vi "Main.vi"() -> ()   [LabVIEW 2018] (continued)
            n624 = Index Array(array=w4544, index (row)=w4543, index (col)=w4543) -> (element=w4542:string)
            n625 = Equal?(x=w4542, y="T") -> (x = y?=w4540:bool)
            n626 = local read "ST102数据"() -> (w4537:string[])
            n627 = case shown="真" w4540 {
              tunnel: w4537 -> [w4577 w4583]
              tunnel: [w4573 w4580] -> w4552
              tunnel: w4536 -> [w4572 w4582]
              tunnel: w4545 -> [w4571 w4581]
              tunnel: w4539 -> [w4570 w4594]
              tunnel: w4538 -> [w4569 w4593]
              tunnel: [w4567 w4579] -> w4534
              frame False {
                n628 = call "SQL_Update.vi"("查询语句"=w4571, "表名"="Online", "error in (no error)"=w4569, "列名对应的值"=w4577, "列名"=string[] ["Last_Station", "Last_Result", "ST10_R_Date", "ST10_R_Time", "ST10_Result", "ST10_Pressure_Final", "ST10_Pressure_Upper", "ST10_Pressure_Lower", "ST10_Displacement_Final", "ST10_Displacement_Upper", "ST10_Displacement_Lower", "ST10_Inflextion_Point", "ST10_Inflextion_Point_Upper", "ST10_Inflextion_Point_Lower", "Grade", "ST10_Sleeve_5020001", "ST10_Flange_5025570"], "connection reference"=w4570) -> ("error out"=w4573:errorcluster)  [unwired: 4 in, 1 out]
                n629 = Unbundle By Name(w4573) -> ("status"=w4576:bool)
                n630 = Equal?(x=w4572, y="") -> (x = y?=w4574:bool)
                n631 = Or(x=w4576, y=w4574) -> (x .or. y?=w4567:bool)
              }
              frame True {
                w4589 = 0 ("索引 (行)")
                n632 = call "SQL_Select.vi"("要读取的列名"=string[] ["[102]"], "表名"="Rework_List", "error in (no error)"=w4593, "查询语句"=w4581, "查询条件"=TRUE, "connection reference"=w4594) -> ("error out"=w4584:errorcluster, "数据"=w4590:string[][], "connection reference out"=w4585:T5)  [unwired: 3 in]
                n633 = Index Array(array=w4590, index (row)=w4589, index (col)=w4589) -> (element=w4588:string)
                n634 = Equal?(x=w4588, y="T") -> (x = y?=w4586:bool)
                n635 = case shown="假" w4586 {
                  tunnel: w4585 -> [w4602 w4618]
                  tunnel: w4584 -> [w4603 w4617]
                  tunnel: w4583 -> [w4601 w4624]
                  tunnel: w4582 -> [w4598 w4619]
                  tunnel: w4581 -> [w4600 w4611]
                  tunnel: [w4599 w4610] -> w4580
                  tunnel: [w4596 w4608] -> w4579
                  frame False {
                    n636 = call "SQL_Update.vi"("查询语句"=w4600, "表名"="Online", "error in (no error)"=w4603, "列名对应的值"=w4601, "列名"=string[] ["Last_Station", "Last_Result", "ST10_R_Date", "ST10_R_Time", "ST10_Result", "ST10_Pressure_Final", "ST10_Pressure_Upper", "ST10_Pressure_Lower", "ST10_Displacement_Final", "ST10_Displacement_Upper", "ST10_Displacement_Lower", "ST10_Inflextion_Point", "ST10_Inflextion_Point_Upper", "ST10_Inflextion_Point_Lower", "Grade", "ST10_Sleeve_5020001", "ST10_Flange_5025570"], "connection reference"=w4602) -> ("error out"=w4599:errorcluster)  [unwired: 4 in, 1 out]
                    n637 = Unbundle By Name(w4599) -> ("status"=w4606:bool)
                    n638 = Equal?(x=w4598, y="") -> (x = y?=w4604:bool)
                    n639 = Or(x=w4606, y=w4604) -> (x .or. y?=w4596:bool)
                  }
                  frame True {
                    n640 = Delete From Array(array=w4624, length=2 ("长度"), index=0 ("索引")) -> (deleted portion=w4612:string[], array with subset deleted=w4621:string[])
                    n641 = call "SQL_Update.vi"("查询语句"=w4611, "表名"="Online", "error in (no error)"=w4617, "列名对应的值"=w4612, "列名"=string[] ["Last_Station", "Last_Result"], "connection reference"=w4618) -> ("error out"=w4616:errorcluster, "connection reference 2"=w4615:T5)  [unwired: 4 in]
                    n642 = call "SQL_Update.vi"("查询语句"=w4611, "表名"="Rework", "error in (no error)"=w4616, "列名对应的值"=w4621, "列名"=string[] ["ST10_R_Date", "ST10_R_Time", "ST10_Result", "ST10_Pressure_Final", "ST10_Pressure_Upper", "ST10_Pressure_Lower", "ST10_Displacement_Final", "ST10_Displacement_Upper", "ST10_Displacement_Lower", "ST10_Inflextion_Point", "ST10_Inflextion_Point_Upper", "ST10_Inflextion_Point_Lower", "Grade", "ST10_Sleeve_5020001", "ST10_Flange_5025570"], "connection reference"=w4615) -> ("error out"=w4610:errorcluster)  [unwired: 4 in, 1 out]
                    n643 = Unbundle By Name(w4610) -> ("status"=w4626:bool)
                    n644 = Equal?(x="", y=w4619) -> (x = y?=w4625:bool)
                    n645 = Or(x=w4626, y=w4625) -> (x .or. y?=w4608:bool)
                  }
                }
              }
            }
            n646 = case shown="假" w4534 {
              frame False {
                n647 = property on="ST10画曲线" class="Bool (严格)"("Val(Sgnl)"=TRUE ("值(信号)")) -> ()  [unwired: 2 in, 2 out]
              }
              frame True {
                n648 = local write "102数据回复写入"(TRUE ("102数据回复写入")) -> ()
                "数据保存请求回复102" <- "2" ("数据保存请求回复102")
              }
            }
            n649 = Delete From Array(array=w4537, length=2 ("长度"), index=0 ("索引")) -> (array with subset deleted=w4555:string[])  [unwired: 1 out]
            n650 = Insert Into Array(array=w4555, index=3 ("索引"), new element=w4536) -> (w4553:string[])
            n651 = Insert Into Array(array=string[][] [] ("数组"), index (row)=0 ("索引 (行)"), new element=w4553) -> (w4558:string[][])  [unwired: 1 in]
            n652 = Transpose 2D Array(2D array=w4558) -> (transposed array=w4535:string[][])
            n653 = property on="ST102_DATA" class="MCListbox (严格)"("ItemNames"=w4535) -> ()  [unwired: 2 in, 2 out]
            "ST102数据读取（事件）" <- FALSE ("ST10数据读取（事件）")
          }
          event "ST201扫码请求(事件)": Value Change {
            w4629 = path "D:/op201" ("路径")
            n654 = event-data() -> ()  [unwired: 1 in, 1 out]
            n655 = List Folder(path=w4629) -> (filenames=w4628:string[])  [unwired: 3 in, 3 out]
            n656 = for {
              tunnel: w4628 -> [w4660] mode=indexing
              tunnel: w4629 -> [w4661]
              n657 = Build Path(base path=w4661, name or relative path=w4660) -> (appended path=w4658:path)
              n658 = Delete(path (use dialog)=w4658, entire hierarchy (F)=TRUE ("整个层次结构(F)")) -> ()  [unwired: 3 in, 3 out]
            }
            n659 = local read "201二维码"() -> (w4634:string)
            n660 = Concatenate Strings("Where QRCode='" ("查询语句"), w4634, "'" ("字符串")) -> (w4651:string)
            n661 = call "SQL_Select.vi"("要读取的列名"=string[] ["Last_Station", "Last_Result"], "表名"="Online", "error in (no error)"=w4640, "查询语句"=w4651, "查询条件"=TRUE, "connection reference"=w4639) -> ("error out"=w4637:errorcluster, "数据"=w4650:string[][])  [unwired: 3 in, 1 out]
            n662 = case shown="无错误" w4637 {
              tunnel: w4650 -> [w4669 _]
              tunnel: ["1" ("右扫码请求回复") "2" ("右扫码请求回复")] -> w4630
              tunnel: [w4664 w4671] -> w4633
              tunnel: [w4663 w4671] -> w4632
              tunnel: [TRUE TRUE] -> w4631
              frame No Error {
                n663 = Index Array(array=w4669, index (row)=0 ("索引 (行)")) -> (element=w4666:string[])  [unwired: 1 in]
                n664 = Index Array(array=w4666, index #1=0 ("索引 (行)")) -> (element #1=w4663:string, element #2=w4664:string)  [unwired: 1 in]
              }
              frame Error {
                w4671 = ""
              }
            }
            "上一站号 (201)" <- w4632
            "上一站结果 (201)" <- w4633
            "扫码请求回复201" <- w4630
            n665 = local write "201扫码回复写入"(w4631) -> ()
            n666 = Get Date/Time String(want seconds? (F)=TRUE ("需要秒？(F)")) -> (time string=w4647:string)  [unwired: 2 in, 1 out]
            n667 = Format Date/Time String(time format string (%c)="%Y-%m-%d" ("时间格式字符串(%c)")) -> (date/time string=w4648:string)  [unwired: 2 in]
            n668 = Insert Into Array(array=string[] [] ("数组"), index=0 ("索引"), new element #1=w4648, new element #2=w4647, new element #3=w4634) -> (w4644:string[])
            n669 = Insert Into Array(array=string[][] [] ("数组"), index (row)=0 ("索引 (行)"), new element=w4644) -> (w4641:string[][])  [unwired: 1 in]
            n670 = Transpose 2D Array(2D array=w4641) -> (transposed array=w4638:string[][])
            n671 = property on="ST201_DATA" class="MCListbox (严格)"("ItemNames"=w4638) -> ()  [unwired: 2 in, 2 out]
            "ST201扫码请求(事件)" <- FALSE ("ST20扫码请求(事件)")
          }
          event "ST201数据读取(事件)": Value Change {
            n672 = event-data() -> ()  [unwired: 1 in, 1 out]
            n673 = flat-sequence {
              tunnel: w4677 -> [w4682]
              tunnel: w4678 -> [w4683]
              tunnel: [w4683] -> w4675
              tunnel: [w4682] -> w4674
              tunnel: w4675 -> [w4689]
              tunnel: w4674 -> [w4688]
              tunnel: [w4687] -> w4673
              tunnel: [w4783] -> w4676
              tunnel: w4673 -> [w4783]
              frame #0 {
                "ST201保存中" <- TRUE
              }
              frame #1 {
                w4695 = 0 ("索引 (行)")
                n674 = local read "201二维码"() -> (w4686:string)
                n675 = Concatenate Strings("Where QRCode='" ("查询语句"), w4686, "'" ("字符串")) -> (w4697:string)
                n676 = call "SQL_Select.vi"("要读取的列名"=string[] ["Rework_Status"], "表名"="Online", "error in (no error)"=w4688, "查询语句"=w4697, "查询条件"=TRUE, "connection reference"=w4689) -> ("error out"=w4690:errorcluster, "数据"=w4696:string[][], "connection reference out"=w4691:T5)  [unwired: 3 in]
                n677 = Index Array(array=w4696, index (row)=w4695, index (col)=w4695) -> (element=w4694:string)
                n678 = Equal?(x=w4694, y="T") -> (x = y?=w4692:bool)
                n679 = local read "201数据"() -> (w4685:string[])
                n680 = case shown="真" w4692 {
                  tunnel: w4685 -> [w4725 w4733]
                  tunnel: [w4721 w4730] -> w4687
                  tunnel: w4686 -> [w4720 w4732]
                  tunnel: w4697 -> [w4719 w4731]
                  tunnel: w4691 -> [w4718 w4744]
                  tunnel: w4690 -> [w4717 w4743]
                  tunnel: [w4715 w4729] -> w4684
                  frame False {
                    n681 = call "SQL_Update.vi"("查询语句"=w4719, "表名"="Online", "error in (no error)"=w4717, "列名对应的值"=w4725, "列名"=string[] ["Last_Station", "Last_Result", "ST201_Date", "ST201_Time", "ST201_Result", "ST201_Oil_Pressure_Final", "ST201_Oil_Pressure_Upper", "ST201_Oil_Pressure_Lower", "ST201_Oil_Displacement_Final", "ST201_Oil_Displacement_Upper", "ST201_Oil_Displacement_Lower", "ST201_Oil_Inflexion_Force_Final", "ST201_Oil_Inflexion_Force_Upper", "ST201_Oil_Inflexion_Force_Lower", "ST201_Bearing_Pressure_Final", "ST201_Bearing_Pressure_Upper", "ST201_Bearing_Pressure_Lower", "ST201_Bearing_Displacement_Final", "ST201_Bearing_Displacement_Upper", "ST201_Bearing_Displacement_Lower", "ST201_Bearing_Inflexion_Force_Final", "ST201_Bearing_Inflexion_Force_Upper", "ST201_Bearing_Inflexion_Force_Lower"], "connection reference"=w4718) -> ("error out"=w4721:errorcluster)  [unwired: 4 in, 1 out]
                    n682 = Unbundle By Name(w4721) -> ("status"=w4724:bool)
                    n683 = Equal?(x=w4720, y="") -> (x = y?=w4722:bool)
                    n684 = Or(x=w4724, y=w4722) -> (x .or. y?=w4715:bool)
                    n685 = case shown="假" w4715 {
                      tunnel: ["1" ("数据保存请求回复") "2" ("数据保存请求回复")] -> _
                      frame False {
                      }
                      frame True {
                      }
                    }
                  }
                  frame True {
                    w4739 = 0 ("索引 (行)")
                    n686 = call "SQL_Select.vi"("要读取的列名"=string[] ["[201]"], "表名"="Rework_List", "error in (no error)"=w4743, "查询语句"=w4731, "查询条件"=TRUE, "connection reference"=w4744) -> ("error out"=w4734:errorcluster, "数据"=w4740:string[][], "connection reference out"=w4735:T5)  [unwired: 3 in]
                    n687 = Index Array(array=w4740, index (row)=w4739, index (col)=w4739) -> (element=w4738:string)
                    n688 = Equal?(x=w4738, y="T") -> (x = y?=w4736:bool)
                    n689 = case shown="假" w4736 {
                      tunnel: w4735 -> [w4752 w4770]
                      tunnel: w4734 -> [w4753 w4769]
                      tunnel: w4733 -> [w4751 w4776]
                      tunnel: w4732 -> [w4748 w4771]
                      tunnel: w4731 -> [w4750 w4762]
                      tunnel: [w4749 w4763] -> w4730
                      tunnel: [w4746 w4760] -> w4729
                      frame False {
                        (unwired) TRUE
                        n690 = call "SQL_Update.vi"("查询语句"=w4750, "表名"="Online", "error in (no error)"=w4753, "列名对应的值"=w4751, "列名"=string[] ["Last_Station", "Last_Result", "ST201_Date", "ST201_Time", "ST201_Result", "ST201_Oil_Pressure_Final", "ST201_Oil_Pressure_Upper", "ST201_Oil_Pressure_Lower", "ST201_Oil_Displacement_Final", "ST201_Oil_Displacement_Upper", "ST201_Oil_Displacement_Lower", "ST201_Oil_Inflexion_Force_Final", "ST201_Oil_Inflexion_Force_Upper", "ST201_Oil_Inflexion_Force_Lower", "ST201_Bearing_Pressure_Final", "ST201_Bearing_Pressure_Upper", "ST201_Bearing_Pressure_Lower", "ST201_Bearing_Displacement_Final", "ST201_Bearing_Displacement_Upper", "ST201_Bearing_Displacement_Lower", "ST201_Bearing_Inflexion_Force_Final", "ST201_Bearing_Inflexion_Force_Upper", "ST201_Bearing_Inflexion_Force_Lower"], "connection reference"=w4752) -> ("error out"=w4749:errorcluster)  [unwired: 4 in, 1 out]
                        n691 = Unbundle By Name(w4749) -> ("status"=w4756:bool)
                        n692 = Equal?(x=w4748, y="") -> (x = y?=w4754:bool)
                        n693 = Or(x=w4756, y=w4754) -> (x .or. y?=w4746:bool)
                        n694 = case shown="假" w4746 {
                          tunnel: ["1" ("数据保存请求回复") "2" ("数据保存请求回复")] -> _
                          frame False {
                          }
                          frame True {
                          }
                        }
                      }
                      frame True {
                        n695 = Delete From Array(array=w4776, length=2 ("长度"), index=0 ("索引")) -> (deleted portion=w4764:string[], array with subset deleted=w4773:string[])
                        n696 = call "SQL_Update.vi"("查询语句"=w4762, "表名"="Online", "error in (no error)"=w4769, "列名对应的值"=w4764, "列名"=string[] ["Last_Station", "Last_Result"], "connection reference"=w4770) -> ("error out"=w4768:errorcluster, "connection reference 2"=w4767:T5)  [unwired: 4 in]
                        n697 = call "SQL_Update.vi"("查询语句"=w4762, "表名"="Rework", "error in (no error)"=w4768, "列名对应的值"=w4773, "列名"=string[] ["ST201_Date", "ST201_Time", "ST201_Result", "ST201_Oil_Pressure_Final", "ST201_Oil_Pressure_Upper", "ST201_Oil_Pressure_Lower", "ST201_Oil_Displacement_Final", "ST201_Oil_Displacement_Upper", "ST201_Oil_Displacement_Lower", "ST201_Oil_Inflexion_Force_Final", "ST201_Oil_Inflexion_Force_Upper", "ST201_Oil_Inflexion_Force_Lower", "ST201_Bearing_Pressure_Final", "ST201_Bearing_Pressure_Upper", "ST201_Bearing_Pressure_Lower", "ST201_Bearing_Displacement_Final", "ST201_Bearing_Displacement_Upper", "ST201_Bearing_Displacement_Lower", "ST201_Bearing_Inflexion_Force_Final", "ST201_Bearing_Inflexion_Force_Upper", "ST201_Bearing_Inflexion_Force_Lower"], "connection reference"=w4767) -> ("error out"=w4763:errorcluster)  [unwired: 4 in, 1 out]
                        n698 = Unbundle By Name(w4763) -> ("status"=w4778:bool)
                        n699 = Equal?(x="", y=w4771) -> (x = y?=w4777:bool)
                        n700 = Or(x=w4778, y=w4777) -> (x .or. y?=w4760:bool)
                        n701 = case shown="真" w4760 {
                          tunnel: ["1" ("数据保存请求回复") "2" ("数据保存请求回复")] -> _
                          frame False {
                          }
                          frame True {
                          }
                        }
                      }
                    }
                  }
                }
                n702 = case shown="真" w4684 {
                  frame False {
                    n703 = property on="ST201画曲线" class="Bool (严格)"("Val(Sgnl)"=TRUE ("值(信号)")) -> ()  [unwired: 2 in, 2 out]
                  }
                  frame True {
                    n704 = local write "201数据回复写入"(TRUE ("201数据回复写入")) -> ()
                    "数据保存请求回复201" <- "2" ("数据保存请求回复201")
                  }
                }
                n705 = Delete From Array(array=w4685, length=2 ("长度"), index=0 ("索引")) -> (array with subset deleted=w4706:string[])  [unwired: 1 out]
                n706 = Insert Into Array(array=w4706, index=2 ("索引"), new element=w4686) -> (w4704:string[])
                n707 = Insert Into Array(array=string[][] [] ("数组"), index (row)=0 ("索引 (行)"), new element=w4704) -> (w4709:string[][])  [unwired: 1 in]
                n708 = Transpose 2D Array(2D array=w4709) -> (transposed array=w4703:string[][])
                n709 = property on="ST201_DATA" class="MCListbox (严格)"("ItemNames"=w4703) -> ()  [unwired: 2 in, 2 out]
              }
              frame #2 {
                n710 = local write "ST201保存中"(FALSE) -> ()
              }
            }
            "ST201数据读取(事件)" <- FALSE ("ST20数据读取(事件)")
          }
          event "ST202扫码请求(事件)": Value Change {
            w4786 = "——" ("字符串")
            w4793 = path "D:/op202" ("路径")
            n711 = event-data() -> ()  [unwired: 1 in, 2 out]
            n712 = local read "202二维码"() -> (w4790:string)
            n713 = List Folder(path=w4793) -> (filenames=w4792:string[])  [unwired: 3 in, 3 out]
            n714 = for {
              tunnel: w4792 -> [w4812] mode=indexing
              tunnel: w4793 -> [w4813]
              n715 = Build Path(base path=w4813, name or relative path=w4812) -> (appended path=w4810:path)
              n716 = Delete(path (use dialog)=w4810, entire hierarchy (F)=TRUE ("整个层次结构(F)")) -> ()  [unwired: 3 in, 3 out]
            }
            n717 = Concatenate Strings("Where QRCode='" ("查询语句"), w4790, "'" ("字符串")) -> (w4806:string)
            n718 = call "SQL_Select.vi"("要读取的列名"=string[] ["Last_Station", "Last_Result"], "表名"="Online", "error in (no error)"=w4797, "查询语句"=w4806, "查询条件"=TRUE, "connection reference"=w4798) -> ("error out"=w4804:errorcluster, "数据"=w4805:string[][])  [unwired: 3 in, 1 out]
            n719 = case shown="无错误" w4804 {
              tunnel: w4805 -> [w4821 _]
              tunnel: ["1" ("右扫码请求回复") "2" ("右扫码请求回复")] -> w4787
              tunnel: [w4816 w4823] -> w4788
              tunnel: [w4815 w4823] -> w4789
              tunnel: [TRUE TRUE] -> w4796
              frame No Error {
                n720 = Index Array(array=w4821, index (row)=0 ("索引 (行)")) -> (element=w4818:string[])  [unwired: 1 in]
                n721 = Index Array(array=w4818, index #1=0 ("索引 (行)")) -> (element #1=w4815:string, element #2=w4816:string)  [unwired: 1 in]
              }
              frame Error {
                w4823 = ""
              }
            }
            "上一站号 (202)" <- w4789
            "上一站结果 (202)" <- w4788
            "扫码请求回复202" <- w4787
            n722 = Format Date/Time String(time format string (%c)="%Y-%m-%d_%H-%M-%S" ("时间格式字符串(%c)")) -> (date/time string=w4785:string)  [unwired: 2 in]
            n723 = local write "202扫码回复写入"(w4796) -> ()
            n724 = Concatenate Strings(w4790, w4786, w4789, w4788, w4787, w4786, w4785) -> (w4784:string)
            n725 = disable-structure shown="禁用" {
              disable-tunnel: w4784 -> [w4808 _]
              frame Disabled {
                n726 = call "站点编码更新（年月日）.vi"("当前编码信息"=w4808, "站别"="202-1") -> ()  [unwired: 10 in]
              }
              frame Enabled {
              }
            }
            "ST202扫码请求(事件)" <- FALSE ("ST202扫码请求(事件)")
          }
          event "ST202数据读取(事件)": Value Change {
            n727 = event-data() -> ()  [unwired: 1 in, 2 out]
            n728 = local read "202二维码"() -> (w4827:string)
            n729 = Not Equal?(x=w4827, y="") -> (x != y?=w4825:bool)
            n730 = case shown="真" w4825 {
              tunnel: w4833 -> [_ w4858]
              tunnel: w4832 -> [_ w4857]
              tunnel: [errorcluster {"status"=TRUE, "code"=0, "source"="，二维码为空"} ("error out") w4836] -> w4831
              tunnel: [TRUE w4840] -> w4829
              tunnel: w4827 -> [_ w4849]
              frame False {
              }
              frame True {
                w4869 = 0 ("索引 (行)")
                n731 = local read "202data"() -> (w4844:string[])
                n732 = Concatenate Strings("Where QRCode='" ("查询语句"), w4849, "'" ("字符串")) -> (w4843:string)
                n733 = call "SQL_Select.vi"("要读取的列名"=string[] ["Rework_Status"], "表名"="Online", "error in (no error)"=w4857, "查询语句"=w4843, "查询条件"=TRUE, "connection reference"=w4858) -> ("error out"=w4845:errorcluster, "数据"=w4871:string[][], "connection reference out"=w4842:T5)  [unwired: 3 in]
                n734 = Format Date/Time String(time format string (%c)="%Y-%m-%d_%H-%M-%S" ("时间格式字符串(%c)")) -> (date/time string=w4853:string)  [unwired: 2 in]
                n735 = Index Array(array=w4871, index (row)=w4869, index (col)=w4869) -> (element=w4854:string)
                n736 = Equal?(x=w4854, y="T") -> (x = y?=w4841:bool)
                n737 = flat-sequence {
                  tunnel: w4843 -> [w4884]
                  tunnel: w4842 -> [w4883]
                  tunnel: w4845 -> [w4882]
                  tunnel: w4844 -> [w4881]
                  tunnel: [w4880] -> w4848
                  tunnel: [w4879] -> w4847
                  tunnel: [w4878] -> w4846
                  tunnel: w4841 -> [w4877]
                  tunnel: [w4876] -> w4839
                  tunnel: [w4875] -> w4838
                  tunnel: [w4874] -> w4837
                  tunnel: w4848 -> [w4950]
                  tunnel: w4847 -> [w4952]
                  tunnel: w4846 -> [w4951]
                  tunnel: [w4943] -> w4840
                  tunnel: w4839 -> [w4942]
                  tunnel: w4838 -> [w4939]
                  tunnel: w4837 -> [w4938]
                  tunnel: [w4937] -> w4836
                  frame #0 {
                    n738 = case shown="假" w4877 {
                      tunnel: w4881 -> [w4885 w4901]
                      tunnel: w4884 -> [w4886 w4900]
                      tunnel: w4883 -> [w4892 w4911]
                      tunnel: w4882 -> [w4891 w4910]
                      tunnel: [w4889 w4899] -> w4880
                      tunnel: [w4886 w4898] -> w4879
                      tunnel: [w4888 w4897] -> w4878
                      tunnel: [FALSE w4896] -> w4876
                      tunnel: [w4886 w4895] -> w4875
                      tunnel: [w4885 w4894] -> w4874
                      frame False {
                        n739 = call "SQL_Update.vi"("查询语句"=w4886, "表名"="Online", "error in (no error)"=w4891, "列名对应的值"=w4885, "列名"=string[] ["Last_Station", "Last_Result", "ST202_Date", "ST202_Time", "ST202_Result", "ST202_Pressure_Final", "ST202_Pressure_Upper", "ST202_Pressure_Lower", "ST202_Displacement_Final", "ST202_Displacement_Upper", "ST202_Displacement_Lower", "ST202_Sealing_5026269", "ST202_Flange_5025570", "ST202_Shaft_5020526", "ST202_Ring_5020571", "ST202_Needle_bearing_5020570"], "connection reference"=w4892) -> ("error out"=w4888:errorcluster, "connection reference 2"=w4889:T5)  [unwired: 4 in]
                      }
                      frame True {
                        w4906 = 0 ("索引 (行)")
                        n740 = call "SQL_Select.vi"("要读取的列名"=string[] ["[202]"], "表名"="Rework_List", "error in (no error)"=w4910, "查询语句"=w4900, "查询条件"=TRUE, "connection reference"=w4911) -> ("error out"=w4902:errorcluster, "数据"=w4907:string[][], "connection reference out"=w4903:T5)  [unwired: 3 in]
                        n741 = Index Array(array=w4907, index (row)=w4906, index (col)=w4906) -> (element=w4905:string)
                        n742 = Equal?(x=w4905, y="T") -> (x = y?=w4896:bool)
                        n743 = case shown="真" w4896 {
                          tunnel: w4903 -> [w4918 w4931]
                          tunnel: w4902 -> [w4919 w4930]
                          tunnel: w4901 -> [w4913 w4935]
                          tunnel: w4900 -> [w4914 w4922]
                          tunnel: [w4916 w4924] -> w4899
                          tunnel: [w4914 w4922] -> w4898
                          tunnel: [w4915 w4923] -> w4897
                          tunnel: [w4914 w4922] -> w4895
                          tunnel: [w4913 w4921] -> w4894
                          frame False {
                            n744 = call "SQL_Update.vi"("查询语句"=w4914, "表名"="Online", "error in (no error)"=w4919, "列名对应的值"=w4913, "列名"=string[] ["Last_Station", "Last_Result", "ST202_Date", "ST202_Time", "ST202_Result", "ST202_Pressure_Final", "ST202_Pressure_Upper", "ST202_Pressure_Lower", "ST202_Displacement_Final", "ST202_Displacement_Upper", "ST202_Displacement_Lower", "ST202_Sealing_5026269", "ST202_Flange_5025570", "ST202_Shaft_5020526", "ST202_Ring_5020571", "ST202_Needle_bearing_5020570"], "connection reference"=w4918) -> ("error out"=w4915:errorcluster, "connection reference 2"=w4916:T5)  [unwired: 4 in]
                          }
                          frame True {
                            n745 = Delete From Array(array=w4935, length=2 ("长度"), index=0 ("索引")) -> (deleted portion=w4921:string[], array with subset deleted=w4932:string[])
                            n746 = call "SQL_Update.vi"("查询语句"=w4922, "表名"="Online", "error in (no error)"=w4930, "列名对应的值"=w4921, "列名"=string[] ["Last_Station", "Last_Result"], "connection reference"=w4931) -> ("error out"=w4929:errorcluster, "connection reference 2"=w4928:T5)  [unwired: 4 in]
                            n747 = call "SQL_Update.vi"("查询语句"=w4922, "表名"="Rework", "error in (no error)"=w4929, "列名对应的值"=w4932, "列名"=string[] ["ST202_Date", "ST202_Time", "ST202_Result", "ST202_Pressure_Final", "ST202_Pressure_Upper", "ST202_Pressure_Lower", "ST202_Displacement_Final", "ST202_Displacement_Upper", "ST202_Displacement_Lower", "ST202_Sealing_5026269", "ST202_Flange_5025570", "ST202_Shaft_5020526", "ST202_Ring_5020571", "ST202_Needle_bearing_5020570"], "connection reference"=w4928) -> ("error out"=w4923:errorcluster, "connection reference 2"=w4924:T5)  [unwired: 4 in]
                          }
                        }
                      }
                    }
                  }
                  frame #1 {
                    w4947 = 0 ("索引 (行)")
                    n748 = call "SQL_Select.vi"("要读取的列名"=string[] ["Last_Station"], "表名"="Online", "error in (no error)"=w4951, "查询语句"=w4952, "查询条件"=TRUE, "connection reference"=w4950) -> ("error out"=w4940:errorcluster, "数据"=w4948:string[][], "connection reference out"=w4941:T5)  [unwired: 3 in]
                    n749 = Index Array(array=w4948, index (row)=w4947) -> (element=w4949:string[])  [unwired: 1 in]
                    n750 = Index Array(array=w4949, index=w4947) -> (element=w4946:string)
                    n751 = Equal?(x=w4946, y="202") -> (x = y?=w4944:bool)
                    n752 = case shown="真" w4944 {
                      tunnel: [w4956 FALSE] -> w4943
                      tunnel: w4942 -> [w4973 _]
                      tunnel: w4941 -> [w4972 _]
                      tunnel: w4940 -> [w4971 _]
                      tunnel: w4939 -> [w4970 _]
                      tunnel: w4938 -> [w4969 _]
                      tunnel: [w4957 errorcluster {"status"=FALSE, "code"=0, "source"=""} ("error out")] -> w4937
                      frame False {
                        w4963 = 0 ("索引 (行)")
                        n753 = case shown="真" w4973 {
                          tunnel: w4972 -> [w4979 w4992]
                          tunnel: w4971 -> [w4980 w4991]
                          tunnel: w4969 -> [w4978 w4996]
                          tunnel: w4970 -> [w4974 w4983]
                          tunnel: [w4976 w4984] -> w4960
                          tunnel: [w4974 w4983] -> w4958
                          tunnel: [w4975 w4982] -> w4959
                          frame False {
                            n754 = call "SQL_Update.vi"("查询语句"=w4974, "表名"="Online", "error in (no error)"=w4980, "列名对应的值"=w4978, "列名"=string[] ["Last_Station", "Last_Result", "ST202_Date", "ST202_Time", "ST202_Result", "ST202_Pressure_Final", "ST202_Pressure_Upper", "ST202_Pressure_Lower", "ST202_Displacement_Final", "ST202_Displacement_Upper", "ST202_Displacement_Lower", "ST202_Sealing_5026269", "ST202_Flange_5025570", "ST202_Shaft_5020526", "ST202_Ring_5020571", "ST202_Needle_bearing_5020570"], "connection reference"=w4979) -> ("error out"=w4975:errorcluster, "connection reference 2"=w4976:T5)  [unwired: 4 in]
                          }
                          frame True {
                            n755 = Delete From Array(array=w4996, length=2 ("长度"), index=0 ("索引")) -> (deleted portion=w4986:string[], array with subset deleted=w4993:string[])
                            n756 = call "SQL_Update.vi"("查询语句"=w4983, "表名"="Online", "error in (no error)"=w4991, "列名对应的值"=w4986, "列名"=string[] ["Last_Station", "Last_Result"], "connection reference"=w4992) -> ("error out"=w4990:errorcluster, "connection reference 2"=w4989:T5)  [unwired: 4 in]
                            n757 = call "SQL_Update.vi"("查询语句"=w4983, "表名"="Rework", "error in (no error)"=w4990, "列名对应的值"=w4993, "列名"=string[] ["ST202_Date", "ST202_Time", "ST202_Result", "ST202_Pressure_Final", "ST202_Pressure_Upper", "ST202_Pressure_Lower", "ST202_Displacement_Final", "ST202_Displacement_Upper", "ST202_Displacement_Lower", "ST202_Sealing_5026269", "ST202_Flange_5025570", "ST202_Shaft_5020526", "ST202_Ring_5020571", "ST202_Needle_bearing_5020570"], "connection reference"=w4989) -> ("error out"=w4982:errorcluster, "connection reference 2"=w4984:T5)  [unwired: 4 in]
                          }
                        }
                        n758 = call "SQL_Select.vi"("要读取的列名"=string[] ["Last_Station"], "表名"="Online", "error in (no error)"=w4959, "查询语句"=w4958, "查询条件"=TRUE, "connection reference"=w4960) -> ("error out"=w4957:errorcluster, "数据"=w4964:string[][])  [unwired: 3 in, 1 out]
                        n759 = Index Array(array=w4964, index (row)=w4963) -> (element=w4965:string[])  [unwired: 1 in]
                        n760 = Index Array(array=w4965, index=w4963) -> (element=w4962:string)
                        n761 = Not Equal?(x=w4962, y="202") -> (x != y?=w4956:bool)
                      }
                      frame True {
                      }
                    }
                  }
                }
                n762 = Concatenate Strings(w4849, "——" ("字符串"), w4854, w4853) -> (w4852:string)
                n763 = disable-structure shown="禁用" {
                  disable-tunnel: w4852 -> [w5000 _]
                  frame Disabled {
                    n764 = call "站点编码更新（年月日）.vi"("当前编码信息"=w5000, "站别"="202-2") -> ()  [unwired: 10 in]
                  }
                  frame Enabled {
                  }
                }
                n765 = Delete From Array(array=w4844, length=2 ("长度"), index=0 ("索引")) -> (array with subset deleted=w4873:string[])  [unwired: 1 out]
                n766 = Insert Into Array(array=w4873, index=2 ("索引"), new element=w4849) -> (w4872:string[])
                n767 = Insert Into Array(array=string[][] [] ("数组"), index (row)=0 ("索引 (行)"), new element=w4872) -> (w4851:string[][])  [unwired: 1 in]
                n768 = Transpose 2D Array(2D array=w4851) -> (transposed array=w4850:string[][])
                n769 = property on="ST202_DATA" class="MCListbox (严格)"("ItemNames"=w4850) -> ()  [unwired: 2 in, 2 out]
              }
            }
            n770 = case shown="真" w4829 {
              frame False {
                n771 = property on="ST202画曲线" class="Bool (严格)"("Val(Sgnl)"=TRUE ("值(信号)")) -> ()  [unwired: 2 in, 2 out]
              }
              frame True {
                n772 = flat-sequence {
                  frame #0 {
                    "数据保存请求回复202" <- "2" ("数据保存请求回复202")
                  }
                  frame #1 {
                    n773 = local write "202数据回复写入"(TRUE ("202数据回复写入")) -> ()
                  }
                }
              }
            }
            "ST202数据读取(事件)" <- FALSE ("ST202数据读取(事件)")
          }
          event "ST301扫码请求 (事件)": Value Change {
            n774 = event-data() -> ()  [unwired: 1 in, 1 out]
            n775 = local read "301二维码"() -> (w5007:string)
            n776 = Concatenate Strings("Where QRCode='" ("查询语句"), w5007, "'" ("字符串")) -> (w5024:string)
            n777 = call "SQL_Select.vi"("要读取的列名"=string[] ["Last_Station", "Last_Result"], "表名"="Online", "error in (no error)"=w5012, "查询语句"=w5024, "查询条件"=TRUE, "connection reference"=w5013) -> ("error out"=w5010:errorcluster, "数据"=w5023:string[][])  [unwired: 3 in, 1 out]
            n778 = case shown="无错误" w5010 {
              tunnel: w5023 -> [w5038 _]
              tunnel: ["1" ("右扫码请求回复") "2" ("右扫码请求回复")] -> w5006
              tunnel: [TRUE TRUE] -> w5005
              frame No Error {
                n779 = Index Array(array=w5038, index (row)=0 ("索引 (行)")) -> (element=w5035:string[])  [unwired: 1 in]
                n780 = Index Array(array=w5035, index #1=0 ("索引 (行)")) -> (element #1=→"上一站号 (301)":string, element #2=→"上一站结果 (301)":string)  [unwired: 1 in]
              }
              frame Error {
              }
            }
            "扫码请求回复301" <- w5006
            n781 = local write "301扫码回复输入"(w5005) -> ()
            n782 = Format Date/Time String(time format string (%c)="%Y-%m-%d" ("时间格式字符串(%c)")) -> (date/time string=w5021:string)  [unwired: 2 in]
            n783 = Get Date/Time String(want seconds? (F)=TRUE ("需要秒？(F)")) -> (time string=w5020:string)  [unwired: 2 in, 1 out]
            n784 = Insert Into Array(array=string[] [] ("数组"), index=0 ("索引"), new element #1=w5021, new element #2=w5020, new element #3=w5007) -> (w5017:string[])
            n785 = Insert Into Array(array=string[][] [] ("数组"), index (row)=0 ("索引 (行)"), new element=w5017) -> (w5014:string[][])  [unwired: 1 in]
            n786 = Transpose 2D Array(2D array=w5014) -> (transposed array=w5011:string[][])
            n787 = property on="ST301_DATA" class="MCListbox (严格)"("ItemNames"=w5011) -> ()  [unwired: 2 in, 2 out]
            "ST301扫码请求 (事件)" <- FALSE ("ST30扫码请求 (事件)")
          }
          event "ST301数据读取 (事件)": Value Change {
            w5053 = 0 ("索引 (行)")
            n788 = event-data() -> ()  [unwired: 1 in, 1 out]
            n789 = local read "301二维码"() -> (w5045:string)
            n790 = Concatenate Strings("Where QRCode='" ("查询语句"), w5045, "'" ("字符串")) -> (w5055:string)
            n791 = call "SQL_Select.vi"("要读取的列名"=string[] ["Rework_Status"], "表名"="Online", "error in (no error)"=w5047, "查询语句"=w5055, "查询条件"=TRUE, "connection reference"=w5046) -> ("error out"=w5048:errorcluster, "数据"=w5054:string[][], "connection reference out"=w5049:T5)  [unwired: 3 in]
            n792 = Index Array(array=w5054, index (row)=w5053, index (col)=w5053) -> (element=w5052:string)
            n793 = Equal?(x=w5052, y="T") -> (x = y?=w5050:bool)
            n794 = local read "301数据"() -> (w5043:string[])
            n795 = case shown="真" w5050 {
              tunnel: [w5084 w5090] -> w5042
              tunnel: w5043 -> [w5083 w5093]
              tunnel: [w5078 w5089] -> w5044
              tunnel: w5045 -> [w5077 w5092]
              tunnel: w5055 -> [w5076 w5091]
              tunnel: w5049 -> [w5075 w5104]
              tunnel: w5048 -> [w5074 w5103]
              tunnel: [TRUE w5088] -> w5041
              frame False {
                n796 = call "SQL_Update.vi"("查询语句"=w5076, "表名"="Online", "error in (no error)"=w5074, "列名对应的值"=w5083, "列名"=string[] ["Last_Station", "Last_Result", "ST301_Date", "ST301_Time", "ST301_Shield", "ST301_Result", "ST301_Magnetic_flux_Left", "ST301_Magnetic_flux_Right", "ST301_Magnetic_flux_Upper", "ST301_Magnetic_flux_Lower", "ST301_PanelNumber"], "connection reference"=w5075) -> ("error out"=w5078:errorcluster)  [unwired: 4 in, 1 out]
                n797 = Unbundle By Name(w5078) -> ("status"=w5082:bool)
                n798 = Equal?(x=w5077, y="") -> (x = y?=w5080:bool)
                n799 = Or(x=w5082, y=w5080) -> (x .or. y?=w5079:bool)
                n800 = case shown="假" w5079 {
                  tunnel: ["1" ("数据保存请求回复") "2" ("数据保存请求回复")] -> w5084
                  frame False {
                  }
                  frame True {
                  }
                }
              }
              frame True {
                w5099 = 0 ("索引 (行)")
                n801 = call "SQL_Select.vi"("要读取的列名"=string[] ["[301]"], "表名"="Rework_List", "error in (no error)"=w5103, "查询语句"=w5091, "查询条件"=TRUE, "connection reference"=w5104) -> ("error out"=w5094:errorcluster, "数据"=w5100:string[][], "connection reference out"=w5095:T5)  [unwired: 3 in]
                n802 = Index Array(array=w5100, index (row)=w5099, index (col)=w5099) -> (element=w5098:string)
                n803 = Equal?(x=w5098, y="T") -> (x = y?=w5096:bool)
                n804 = case shown="真" w5096 {
                  tunnel: w5095 -> [w5113 w5133]
                  tunnel: w5094 -> [w5114 w5132]
                  tunnel: w5093 -> [w5112 w5139]
                  tunnel: w5092 -> [w5109 w5134]
                  tunnel: w5091 -> [w5111 w5124]
                  tunnel: [w5108 w5126] -> w5090
                  tunnel: [w5110 w5125] -> w5089
                  tunnel: [TRUE TRUE] -> w5088
                  frame False {
                    n805 = call "SQL_Update.vi"("查询语句"=w5111, "表名"="Online", "error in (no error)"=w5114, "列名对应的值"=w5112, "列名"=string[] ["Last_Station", "Last_Result", "ST301_Date", "ST301_Time", "ST301_Shield", "ST301_Result", "ST301_Magnetic_flux_Left", "ST301_Magnetic_flux_Right", "ST301_Magnetic_flux_Upper", "ST301_Magnetic_flux_Lower", "ST301_PanelNumber"], "connection reference"=w5113) -> ("error out"=w5110:errorcluster)  [unwired: 4 in, 1 out]
                    n806 = Unbundle By Name(w5110) -> ("status"=w5118:bool)
                    n807 = Equal?(x=w5109, y="") -> (x = y?=w5116:bool)
                    n808 = Or(x=w5118, y=w5116) -> (x .or. y?=w5115:bool)
                    n809 = case shown="假" w5115 {
                      tunnel: ["1" ("数据保存请求回复") "2" ("数据保存请求回复")] -> w5108
                      frame False {
                      }
                      frame True {
                      }
                    }
                  }
                  frame True {
                    n810 = Delete From Array(array=w5139, length=2 ("长度"), index=0 ("索引")) -> (deleted portion=w5127:string[], array with subset deleted=w5136:string[])
                    n811 = call "SQL_Update.vi"("查询语句"=w5124, "表名"="Online", "error in (no error)"=w5132, "列名对应的值"=w5127, "列名"=string[] ["Last_Station", "Last_Result"], "connection reference"=w5133) -> ("error out"=w5131:errorcluster, "connection reference 2"=w5130:T5)  [unwired: 4 in]
                    n812 = call "SQL_Update.vi"("查询语句"=w5124, "表名"="Rework", "error in (no error)"=w5131, "列名对应的值"=w5136, "列名"=string[] ["ST301_Date", "ST301_Time", "ST301_Shield", "ST301_Result", "ST301_Magnetic_flux_Left", "ST301_Magnetic_flux_Right", "ST301_Magnetic_flux_Upper", "ST301_Magnetic_flux_Lower", "ST301_PanelNumber"], "connection reference"=w5130) -> ("error out"=w5125:errorcluster)  [unwired: 4 in, 1 out]
                    n813 = Unbundle By Name(w5125) -> ("status"=w5142:bool)
                    n814 = Equal?(x="", y=w5134) -> (x = y?=w5141:bool)
                    n815 = Or(x=w5142, y=w5141) -> (x .or. y?=w5140:bool)
                    n816 = case shown="真" w5140 {
                      tunnel: ["1" ("数据保存请求回复") "2" ("数据保存请求回复")] -> w5126
                      frame False {
                      }
                      frame True {
                      }
                    }
                  }
                }
              }
            }
            "数据保存请求回复301" <- w5042
            n817 = local write "301数据回复输入"(w5041) -> ()
            n818 = Delete From Array(array=w5043, length=2 ("长度"), index=0 ("索引")) -> (array with subset deleted=w5065:string[])  [unwired: 1 out]
            n819 = Insert Into Array(array=w5065, index=2 ("索引"), new element=w5045) -> (w5063:string[])
            n820 = Insert Into Array(array=string[][] [] ("数组"), index (row)=0 ("索引 (行)"), new element=w5063) -> (w5068:string[][])  [unwired: 1 in]
            n821 = Transpose 2D Array(2D array=w5068) -> (transposed array=w5062:string[][])
            n822 = property on="ST301_DATA" class="MCListbox (严格)"("ItemNames"=w5062) -> ()  [unwired: 2 in, 2 out]
            "ST301数据读取 (事件)" <- FALSE ("ST30数据读取 (事件)")
          }
          event "ST302扫码请求 (事件)": Value Change {
            n823 = event-data() -> ()  [unwired: 1 in, 2 out]
            n824 = local read "302二维码"() -> (w5149:string)
            n825 = Concatenate Strings("Where QRCode='" ("查询语句"), w5149, "'" ("字符串")) -> (w5159:string)
            n826 = call "SQL_Select.vi"("要读取的列名"=string[] ["Last_Station", "Last_Result"], "表名"="Online", "error in (no error)"=w5151, "查询语句"=w5159, "查询条件"=TRUE, "connection reference"=w5152) -> ("error out"=w5150:errorcluster, "数据"=w5158:string[][])  [unwired: 3 in, 1 out]
            n827 = case shown="无错误" w5150 {
              tunnel: w5158 -> [w5168 _]
              tunnel: ["1" ("右扫码请求回复") "2" ("右扫码请求回复")] -> w5148
              tunnel: [TRUE TRUE] -> w5147
              frame No Error {
                n828 = Index Array(array=w5168, index (row)=0 ("索引 (行)")) -> (element=w5165:string[])  [unwired: 1 in]
                n829 = Index Array(array=w5165, index #1=0 ("索引 (行)")) -> (element #1=→"上一站号 (302)":string, element #2=→"上一站结果 (302)":string)  [unwired: 1 in]
              }
              frame Error {
              }
            }
            "扫码请求回复302" <- w5148
            n830 = local write "302扫码回复输入"(w5147) -> ()
            "ST302扫码请求 (事件)" <- FALSE ("ST302扫码请求 (事件)")
          }
          event "ST302数据读取 (事件)": Value Change {
            w5190 = 0 ("索引 (行)")
            n831 = event-data() -> ()  [unwired: 1 in, 2 out]
            n832 = local read "302二维码"() -> (w5177:string)
            n833 = Concatenate Strings("Where QRCode='" ("查询语句"), w5177, "'" ("字符串")) -> (w5197:string)
            n834 = call "SQL_Select.vi"("要读取的列名"=string[] ["Rework_Status"], "表名"="Online", "error in (no error)"=w5178, "查询语句"=w5197, "查询条件"=TRUE, "connection reference"=w5179) -> ("error out"=w5192:errorcluster, "数据"=w5196:string[][], "connection reference out"=w5193:T5)  [unwired: 3 in]
            n835 = Index Array(array=w5196, index (row)=w5190, index (col)=w5190) -> (element=w5195:string)
            n836 = Equal?(x=w5195, y="T") -> (x = y?=w5194:bool)
            n837 = local read "302data"() -> (w5176:string[])
            n838 = case shown="真" w5194 {
              tunnel: [w5214 w5220] -> w5175
              tunnel: w5176 -> [w5213 w5223]
              tunnel: [w5208 w5219] -> w5173
              tunnel: w5177 -> [w5207 w5222]
              tunnel: w5197 -> [w5206 w5221]
              tunnel: w5193 -> [w5205 w5234]
              tunnel: w5192 -> [w5204 w5233]
              tunnel: [TRUE w5218] -> w5174
              frame False {
                n839 = call "SQL_Update.vi"("查询语句"=w5206, "表名"="Online", "error in (no error)"=w5204, "列名对应的值"=w5213, "列名"=string[] ["Last_Station", "Last_Result", "ST302_Date", "ST302_Time", "ST302_Result", "ST302_PanelNumber"], "connection reference"=w5205) -> ("error out"=w5208:errorcluster)  [unwired: 4 in, 1 out]
                n840 = Unbundle By Name(w5208) -> ("status"=w5212:bool)
                n841 = Equal?(x=w5207, y="") -> (x = y?=w5210:bool)
                n842 = Or(x=w5212, y=w5210) -> (x .or. y?=w5209:bool)
                n843 = case shown="假" w5209 {
                  tunnel: ["1" ("数据保存请求回复") "2" ("数据保存请求回复")] -> w5214
                  frame False {
                  }
                  frame True {
                  }
                }
              }
              frame True {
                w5229 = 0 ("索引 (行)")
                n844 = call "SQL_Select.vi"("要读取的列名"=string[] ["[302]"], "表名"="Rework_List", "error in (no error)"=w5233, "查询语句"=w5221, "查询条件"=TRUE, "connection reference"=w5234) -> ("error out"=w5224:errorcluster, "数据"=w5230:string[][], "connection reference out"=w5225:T5)  [unwired: 3 in]
                n845 = Index Array(array=w5230, index (row)=w5229, index (col)=w5229) -> (element=w5228:string)
                n846 = Equal?(x=w5228, y="T") -> (x = y?=w5226:bool)
                n847 = case shown="真" w5226 {
                  tunnel: w5225 -> [w5243 w5263]
                  tunnel: w5224 -> [w5244 w5262]
                  tunnel: w5223 -> [w5242 w5269]
                  tunnel: w5222 -> [w5239 w5264]
                  tunnel: w5221 -> [w5241 w5254]
                  tunnel: [w5238 w5256] -> w5220
                  tunnel: [w5240 w5255] -> w5219
                  tunnel: [TRUE TRUE] -> w5218
                  frame False {
                    n848 = call "SQL_Update.vi"("查询语句"=w5241, "表名"="Online", "error in (no error)"=w5244, "列名对应的值"=w5242, "列名"=string[] ["Last_Station", "Last_Result", "ST302_Date", "ST302_Time", "ST302_Result", "ST302_PanelNumber"], "connection reference"=w5243) -> ("error out"=w5240:errorcluster)  [unwired: 4 in, 1 out]
                    n849 = Unbundle By Name(w5240) -> ("status"=w5248:bool)
                    n850 = Equal?(x=w5239, y="") -> (x = y?=w5246:bool)
                    n851 = Or(x=w5248, y=w5246) -> (x .or. y?=w5245:bool)
                    n852 = case shown="假" w5245 {
                      tunnel: ["1" ("数据保存请求回复") "2" ("数据保存请求回复")] -> w5238
                      frame False {
                      }
                      frame True {
                      }
                    }
                  }
                  frame True {
                    n853 = Delete From Array(array=w5269, length=2 ("长度"), index=0 ("索引")) -> (deleted portion=w5257:string[], array with subset deleted=w5266:string[])
                    n854 = call "SQL_Update.vi"("查询语句"=w5254, "表名"="Online", "error in (no error)"=w5262, "列名对应的值"=w5257, "列名"=string[] ["Last_Station", "Last_Result"], "connection reference"=w5263) -> ("error out"=w5261:errorcluster, "connection reference 2"=w5260:T5)  [unwired: 4 in]
                    n855 = call "SQL_Update.vi"("查询语句"=w5254, "表名"="Rework", "error in (no error)"=w5261, "列名对应的值"=w5266, "列名"=string[] ["ST302_Date", "ST302_Time", "ST302_Result", "ST302_PanelNumber"], "connection reference"=w5260) -> ("error out"=w5255:errorcluster)  [unwired: 4 in, 1 out]
                    n856 = Unbundle By Name(w5255) -> ("status"=w5272:bool)
                    n857 = Equal?(x="", y=w5264) -> (x = y?=w5271:bool)
                    n858 = Or(x=w5272, y=w5271) -> (x .or. y?=w5270:bool)
                    n859 = case shown="真" w5270 {
                      tunnel: ["1" ("数据保存请求回复") "2" ("数据保存请求回复")] -> w5256
                      frame False {
                      }
                      frame True {
                      }
                    }
                  }
                }
              }
            }
            "数据保存请求回复302" <- w5175
            n860 = local write "302数据回复输入"(w5174) -> ()
            n861 = Delete From Array(array=w5176, length=2 ("长度"), index=0 ("索引")) -> (array with subset deleted=w5199:string[])  [unwired: 1 out]
            n862 = Insert Into Array(array=w5199, index=2 ("索引"), new element=w5177) -> (w5198:string[])
            n863 = Insert Into Array(array=string[][] [] ("数组"), index (row)=0 ("索引 (行)"), new element=w5198) -> (w5200:string[][])  [unwired: 1 in]
            n864 = Transpose 2D Array(2D array=w5200) -> (transposed array=w5171:string[][])
            n865 = property on="ST302_DATA" class="MCListbox (严格)"("ItemNames"=w5171) -> ()  [unwired: 2 in, 2 out]
            "ST302数据读取 (事件)" <- FALSE ("ST302数据读取 (事件)")
          }
          event "ST303扫码请求 (事件)": Value Change {
            n866 = event-data() -> ()  [unwired: 1 in, 2 out]
            n867 = local read "303二维码"() -> (w5278:string)
            n868 = Concatenate Strings("Where QRCode='" ("查询语句"), w5278, "'" ("字符串")) -> (w5289:string)
            n869 = call "SQL_Select.vi"("要读取的列名"=string[] ["Last_Station", "Last_Result"], "表名"="Online", "error in (no error)"=w5281, "查询语句"=w5289, "查询条件"=TRUE, "connection reference"=w5282) -> ("error out"=w5280:errorcluster, "数据"=w5288:string[][])  [unwired: 3 in, 1 out]
            n870 = case shown="无错误" w5280 {
              tunnel: w5288 -> [w5298 _]
              tunnel: ["1" ("右扫码请求回复") "2" ("右扫码请求回复")] -> w5277
              tunnel: [TRUE TRUE] -> w5276
              frame No Error {
                n871 = Index Array(array=w5298, index (row)=0 ("索引 (行)")) -> (element=w5295:string[])  [unwired: 1 in]
                n872 = Index Array(array=w5295, index #1=0 ("索引 (行)")) -> (element #1=→"上一站号 (303)":string, element #2=→"上一站结果 (303)":string)  [unwired: 1 in]
              }
              frame Error {
              }
            }
            "扫码请求回复303" <- w5277
            n873 = local write "303扫码回复输入"(w5276) -> ()
            "ST303扫码请求 (事件)" <- FALSE ("ST303扫码请求 (事件)")
          }
          event "ST303数据读取 (事件)": Value Change {
            w5323 = 0 ("索引 (行)")
            n874 = event-data() -> ()  [unwired: 1 in, 2 out]
            n875 = local read "303二维码"() -> (w5302:string)
            n876 = Concatenate Strings("Where QRCode='" ("查询语句"), w5302, "'" ("字符串")) -> (w5330:string)
            n877 = call "SQL_Select.vi"("要读取的列名"=string[] ["Rework_Status"], "表名"="Online", "error in (no error)"=w5316, "查询语句"=w5330, "查询条件"=TRUE, "connection reference"=w5317) -> ("error out"=w5325:errorcluster, "数据"=w5329:string[][], "connection reference out"=w5326:T5)  [unwired: 3 in]
            n878 = Index Array(array=w5329, index (row)=w5323, index (col)=w5323) -> (element=w5328:string)
            n879 = Equal?(x=w5328, y="T") -> (x = y?=w5327:bool)
            n880 = local read "303data"() -> (w5303:string[])
            n881 = case shown="真" w5327 {
              tunnel: [w5344 w5350] -> w5315
              tunnel: w5303 -> [w5343 w5353]
              tunnel: [w5338 w5349] -> w5313
              tunnel: w5302 -> [w5337 w5352]
              tunnel: w5330 -> [w5336 w5351]
              tunnel: w5326 -> [w5335 w5364]
              tunnel: w5325 -> [w5334 w5363]
              tunnel: [TRUE w5348] -> w5314
              frame False {
                n882 = call "SQL_Update.vi"("查询语句"=w5336, "表名"="Online", "error in (no error)"=w5334, "列名对应的值"=w5343, "列名"=string[] ["Last_Station", "Last_Result", "ST303_Date", "ST303_Time", "ST303_Result", "ST303_PanelNumber", "ST303_Cam_ring_5020689", "ST303_Pin_5026280", "ST303_Rotor_5018111"], "connection reference"=w5335) -> ("error out"=w5338:errorcluster)  [unwired: 4 in, 1 out]
                n883 = Unbundle By Name(w5338) -> ("status"=w5342:bool)
                n884 = Equal?(x=w5337, y="") -> (x = y?=w5340:bool)
                n885 = Or(x=w5342, y=w5340) -> (x .or. y?=w5339:bool)
                n886 = case shown="假" w5339 {
                  tunnel: ["1" ("数据保存请求回复") "2" ("数据保存请求回复")] -> w5344
                  frame False {
                  }
                  frame True {
                  }
                }
              }
              frame True {
                w5359 = 0 ("索引 (行)")
                n887 = call "SQL_Select.vi"("要读取的列名"=string[] ["[303]"], "表名"="Rework_List", "error in (no error)"=w5363, "查询语句"=w5351, "查询条件"=TRUE, "connection reference"=w5364) -> ("error out"=w5354:errorcluster, "数据"=w5360:string[][], "connection reference out"=w5355:T5)  [unwired: 3 in]
                n888 = Index Array(array=w5360, index (row)=w5359, index (col)=w5359) -> (element=w5358:string)
                n889 = Equal?(x=w5358, y="T") -> (x = y?=w5356:bool)
                n890 = case shown="真" w5356 {
                  tunnel: w5355 -> [w5373 w5393]
                  tunnel: w5354 -> [w5374 w5392]
                  tunnel: w5353 -> [w5372 w5399]
                  tunnel: w5352 -> [w5369 w5394]
                  tunnel: w5351 -> [w5371 w5384]
                  tunnel: [w5368 w5386] -> w5350
                  tunnel: [w5370 w5385] -> w5349
                  tunnel: [TRUE TRUE] -> w5348
                  frame False {
                    n891 = call "SQL_Update.vi"("查询语句"=w5371, "表名"="Online", "error in (no error)"=w5374, "列名对应的值"=w5372, "列名"=string[] ["Last_Station", "Last_Result", "ST303_Date", "ST303_Time", "ST303_Result", "ST303_PanelNumber", "ST303_Cam_ring_5020689", "ST303_Pin_5026280", "ST303_Rotor_5018111"], "connection reference"=w5373) -> ("error out"=w5370:errorcluster)  [unwired: 4 in, 1 out]
                    n892 = Unbundle By Name(w5370) -> ("status"=w5378:bool)
                    n893 = Equal?(x=w5369, y="") -> (x = y?=w5376:bool)
                    n894 = Or(x=w5378, y=w5376) -> (x .or. y?=w5375:bool)
                    n895 = case shown="假" w5375 {
                      tunnel: ["1" ("数据保存请求回复") "2" ("数据保存请求回复")] -> w5368
                      frame False {
                      }
                      frame True {
                      }
                    }
                  }
                  frame True {
                    n896 = Delete From Array(array=w5399, length=2 ("长度"), index=0 ("索引")) -> (deleted portion=w5387:string[], array with subset deleted=w5396:string[])
                    n897 = call "SQL_Update.vi"("查询语句"=w5384, "表名"="Online", "error in (no error)"=w5392, "列名对应的值"=w5387, "列名"=string[] ["Last_Station", "Last_Result"], "connection reference"=w5393) -> ("error out"=w5391:errorcluster, "connection reference 2"=w5390:T5)  [unwired: 4 in]
                    n898 = call "SQL_Update.vi"("查询语句"=w5384, "表名"="Rework", "error in (no error)"=w5391, "列名对应的值"=w5396, "列名"=string[] ["ST303_Date", "ST303_Time", "ST303_Result", "ST303_PanelNumber", "ST303_Cam_ring_5020689", "ST303_Pin_5026280", "ST303_Rotor_5018111"], "connection reference"=w5390) -> ("error out"=w5385:errorcluster)  [unwired: 4 in, 1 out]
                    n899 = Unbundle By Name(w5385) -> ("status"=w5402:bool)
                    n900 = Equal?(x="", y=w5394) -> (x = y?=w5401:bool)
                    n901 = Or(x=w5402, y=w5401) -> (x .or. y?=w5400:bool)
                    n902 = case shown="真" w5400 {
                      tunnel: ["1" ("数据保存请求回复") "2" ("数据保存请求回复")] -> w5386
                      frame False {
                      }
                      frame True {
                      }
                    }
                  }
                }
              }
            }
            "数据保存请求回复303" <- w5315
            n903 = local write "303数据回复输入"(w5314) -> ()
            n904 = Delete From Array(array=w5303, length=2 ("长度"), index=0 ("索引")) -> (array with subset deleted=w5310:string[])  [unwired: 1 out]
            n905 = Insert Into Array(array=w5310, index=2 ("索引"), new element=w5302) -> (w5309:string[])
            n906 = Insert Into Array(array=string[][] [] ("数组"), index (row)=0 ("索引 (行)"), new element=w5309) -> (w5311:string[][])  [unwired: 1 in]
            n907 = Transpose 2D Array(2D array=w5311) -> (transposed array=w5301:string[][])
            n908 = property on="ST303_DATA" class="MCListbox (严格)"("ItemNames"=w5301) -> ()  [unwired: 2 in, 2 out]
            "ST303数据读取 (事件)" <- FALSE ("ST303数据读取 (事件)")
          }
          event "ST401扫码请求（事件）": Value Change {
            n909 = event-data() -> ()  [unwired: 1 in, 2 out]
            n910 = local read "401二维码"() -> (w5408:string)
            n911 = Concatenate Strings("Where QRCode='" ("查询语句"), w5408, "'" ("字符串")) -> (w5419:string)
            n912 = call "SQL_Select.vi"("要读取的列名"=string[] ["Last_Station", "Last_Result"], "表名"="Online", "error in (no error)"=w5411, "查询语句"=w5419, "查询条件"=TRUE, "connection reference"=w5412) -> ("error out"=w5410:errorcluster, "数据"=w5418:string[][])  [unwired: 3 in, 1 out]
            n913 = case shown="无错误" w5410 {
              tunnel: w5418 -> [w5428 _]
              tunnel: ["1" ("右扫码请求回复") "2" ("右扫码请求回复")] -> w5406
              tunnel: [TRUE TRUE] -> w5407
              frame No Error {
                n914 = Index Array(array=w5428, index (row)=0 ("索引 (行)")) -> (element=w5425:string[])  [unwired: 1 in]
                n915 = Index Array(array=w5425, index #1=0 ("索引 (行)")) -> (element #1=→"上一站号 (401)":string, element #2=→"上一站结果 (401)":string)  [unwired: 1 in]
              }
              frame Error {
              }
            }
            "扫码请求回复401" <- w5406
            n916 = local write "401扫码回复写入"(w5407) -> ()
            "ST401扫码请求（事件）" <- FALSE ("ST401扫码请求（事件）")
          }
          event "ST401数据读取（事件）": Value Change {
            w5453 = 0 ("索引 (行)")
            n917 = event-data() -> ()  [unwired: 1 in, 2 out]
            n918 = local read "401二维码"() -> (w5432:string)
            n919 = Concatenate Strings("Where QRCode='" ("查询语句"), w5432, "'" ("字符串")) -> (w5460:string)
            n920 = call "SQL_Select.vi"("要读取的列名"=string[] ["Rework_Status"], "表名"="Online", "error in (no error)"=w5446, "查询语句"=w5460, "查询条件"=TRUE, "connection reference"=w5447) -> ("error out"=w5455:errorcluster, "数据"=w5459:string[][], "connection reference out"=w5456:T5)  [unwired: 3 in]
            n921 = Index Array(array=w5459, index (row)=w5453, index (col)=w5453) -> (element=w5458:string)
            n922 = Equal?(x=w5458, y="T") -> (x = y?=w5457:bool)
            n923 = local read "401数据"() -> (w5433:string[])
            n924 = case shown="假" w5457 {
              tunnel: [w5474 w5480] -> w5445
              tunnel: w5433 -> [w5473 w5483]
              tunnel: [w5468 w5479] -> w5443
              tunnel: w5432 -> [w5467 w5482]
              tunnel: w5460 -> [w5466 w5481]
              tunnel: w5456 -> [w5465 w5494]
              tunnel: w5455 -> [w5464 w5493]
              tunnel: [TRUE w5478] -> w5444
              frame False {
                n925 = call "SQL_Update.vi"("查询语句"=w5466, "表名"="Online", "error in (no error)"=w5464, "列名对应的值"=w5473, "列名"=string[] ["Last_Station", "Last_Result", "ST401_Date", "ST401_Time", "ST401_Result", "ST401_PanelNumber", "ST401_Shield"], "connection reference"=w5465) -> ("error out"=w5468:errorcluster)  [unwired: 4 in, 1 out]
                n926 = Unbundle By Name(w5468) -> ("status"=w5472:bool)
                n927 = Equal?(x=w5467, y="") -> (x = y?=w5470:bool)
                n928 = Or(x=w5472, y=w5470) -> (x .or. y?=w5469:bool)
                n929 = case shown="假" w5469 {
                  tunnel: ["1" ("数据保存请求回复") "2" ("数据保存请求回复")] -> w5474
                  frame False {
                  }
                  frame True {
                  }
                }
              }
              frame True {
                w5489 = 0 ("索引 (行)")
                n930 = call "SQL_Select.vi"("要读取的列名"=string[] ["[401]"], "表名"="Rework_List", "error in (no error)"=w5493, "查询语句"=w5481, "查询条件"=TRUE, "connection reference"=w5494) -> ("error out"=w5484:errorcluster, "数据"=w5490:string[][], "connection reference out"=w5485:T5)  [unwired: 3 in]
                n931 = Index Array(array=w5490, index (row)=w5489, index (col)=w5489) -> (element=w5488:string)
                n932 = Equal?(x=w5488, y="T") -> (x = y?=w5486:bool)
                n933 = case shown="真" w5486 {
                  tunnel: w5485 -> [w5503 w5523]
                  tunnel: w5484 -> [w5504 w5522]
                  tunnel: w5483 -> [w5502 w5529]
                  tunnel: w5482 -> [w5499 w5524]
                  tunnel: w5481 -> [w5501 w5514]
                  tunnel: [w5498 w5516] -> w5480
                  tunnel: [w5500 w5515] -> w5479
                  tunnel: [TRUE TRUE] -> w5478
                  frame False {
                    n934 = call "SQL_Update.vi"("查询语句"=w5501, "表名"="Online", "error in (no error)"=w5504, "列名对应的值"=w5502, "列名"=string[] ["Last_Station", "Last_Result", "ST401_Date", "ST401_Time", "ST401_Result", "ST401_PanelNumber", "ST401_Shield"], "connection reference"=w5503) -> ("error out"=w5500:errorcluster)  [unwired: 4 in, 1 out]
                    n935 = Unbundle By Name(w5500) -> ("status"=w5508:bool)
                    n936 = Equal?(x=w5499, y="") -> (x = y?=w5506:bool)
                    n937 = Or(x=w5508, y=w5506) -> (x .or. y?=w5505:bool)
                    n938 = case shown="假" w5505 {
                      tunnel: ["1" ("数据保存请求回复") "2" ("数据保存请求回复")] -> w5498
                      frame False {
                      }
                      frame True {
                      }
                    }
                  }
                  frame True {
